vi "MapExample.vi"() -> ()   [LabVIEW 2016]
uses:
  <userlib>/836-libraries/Data_Structures/Map/Map.lvclass
panel:
  out "data":T1
  in  "Cluster":T1
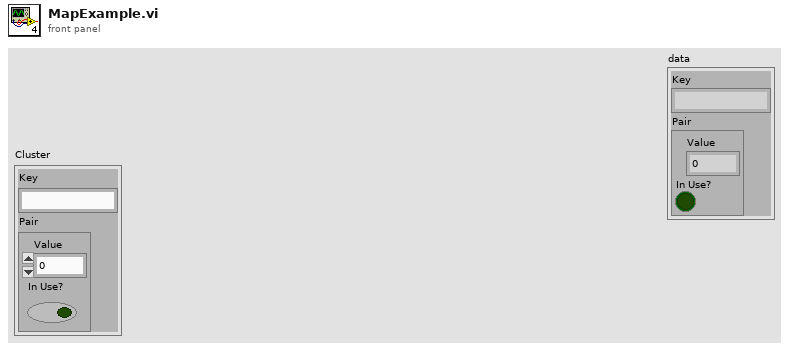
[diagram p1: front panel]
types:
  T1 = cluster{"Key":string, "Pair":cluster{"Value":dbl, "In Use?":bool}}
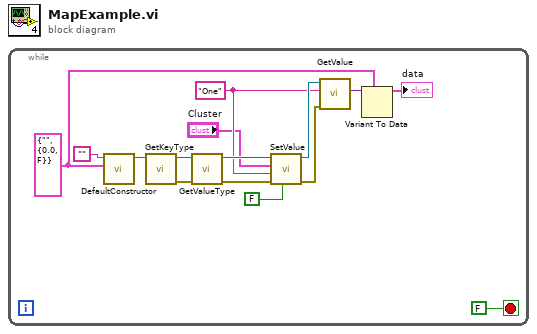
[diagram p0: block diagram]
diagram:
  n1 = while {
    stop <- FALSE stop-if-true
    w3 = T1 {"Key"="", "Pair"={"Value"=0.0, "In Use?"=FALSE}} ("Cluster")
    w7 = "One"
    n2 = call <userlib>:"DefaultConstructor.vi"("ValueType"=w3, "KeyType"="") -> ("Map"=w14:refnum<class "Map.lvclass">)  [unwired: 9 in]
    n3 = call <userlib>:"GetKeyType.vi"("Map in"=w14) -> ("error out"=w9:errorcluster, "Map out"=w13:refnum<class "Map.lvclass">)  [unwired: 8 in, 1 out]
    n4 = call <userlib>:"GetValueType.vi"("error in (no error)"=w9, "Map in"=w13) -> ("error out"=w10:errorcluster, "Map out"=w12:refnum<class "Map.lvclass">)  [unwired: 7 in, 1 out]
    n5 = call <userlib>:"SetValue.vi"("Replace?"=FALSE, "error in (no error)"=w10, "Key"=w7, "Value"="Cluster", "Map in"=w12) -> ("error out"=w6:errorcluster, "Map out"=w8:refnum<class "Map.lvclass">)  [unwired: 3 in, 2 out]
    n6 = call <userlib>:"GetValue.vi"("error in (no error)"=w6, "Key"=w7, "Map in"=w8) -> ("Value"=w5:variant)  [unwired: 5 in, 3 out]
    n7 = Variant To Data(type=w3, Variant=w5) -> (data=→"data":T1)  [unwired: 1 in, 1 out]
  }
